vi "適應性控制_多頻率追蹤DAQmx_V4(實際控制).vi"() -> ()   [LabVIEW 2010]
uses:
  <vilib>/DAQmx/write.llb/DAQmx Write (Analog DBL 1Chan 1Samp).vi
  <vilib>/DAQmx/read.llb/DAQmx Read (Analog DBL 1Chan 1Samp).vi
  <vilib>/DAQmx/create/channels.llb/DAQmx Create Channel (AI-Voltage-Basic).vi
  <vilib>/DAQmx/configure/timing.llb/DAQmx Timing (Sample Clock).vi
  <vilib>/DAQmx/create/channels.llb/DAQmx Create Channel (AO-Voltage-Basic).vi
  <vilib>/daqmx/miscellaneous.llb/DAQmx Fill In Error Info.vi
panel:
  in  "DAQ output":tag
  in  "DAQ input":tag
  out "source out":string
  in  "理想初始頻率(Hz)":dbl=1.0
  in  "理想頻率數":i32=2
  out "當下誤差":dbl=0.1 format="%#_13g"
  out "實際輸入x(t)":dbl[][](graph)
  in  "頻率間距":dbl=1.0
  out "理想與FIR輸出":dbl[][](graph)
  out "誤差":dbl(graph)
  out "while平均運行時間":dbl
  out "收斂time":dbl
  out "各頻率誤差已達標準":bool
  in  "各頻率誤差低於多少亮燈":dbl=0.1 format="%#_13g"
  out "權重(w)":dbl[](array[numeric])
  in  "理想振幅":dbl=0.5
  in  "理想直流偏移":dbl
  in  "理想相位(deg)":dbl
  in  "收斂係數":dbl=0.0001
  in  "order":i32=150
  in  "取樣頻率":dbl=150.0 min=1.0 max=10000.0 step=1.0
  in  "stop":bool
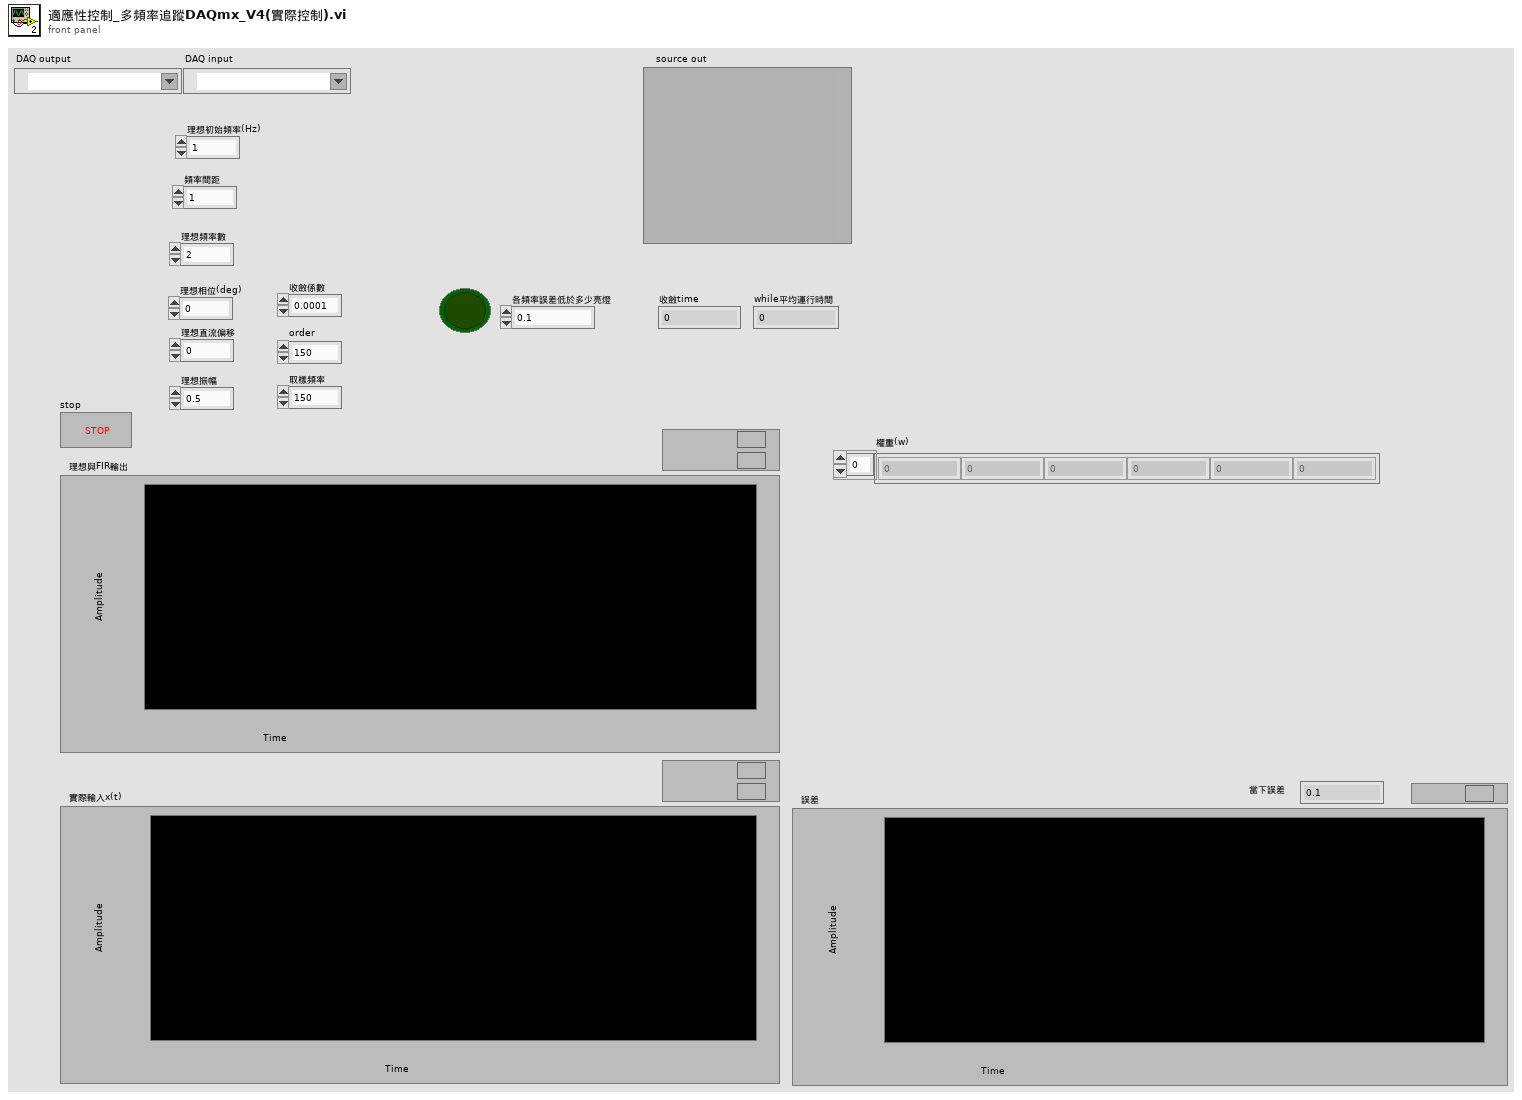
[diagram p1: front panel]
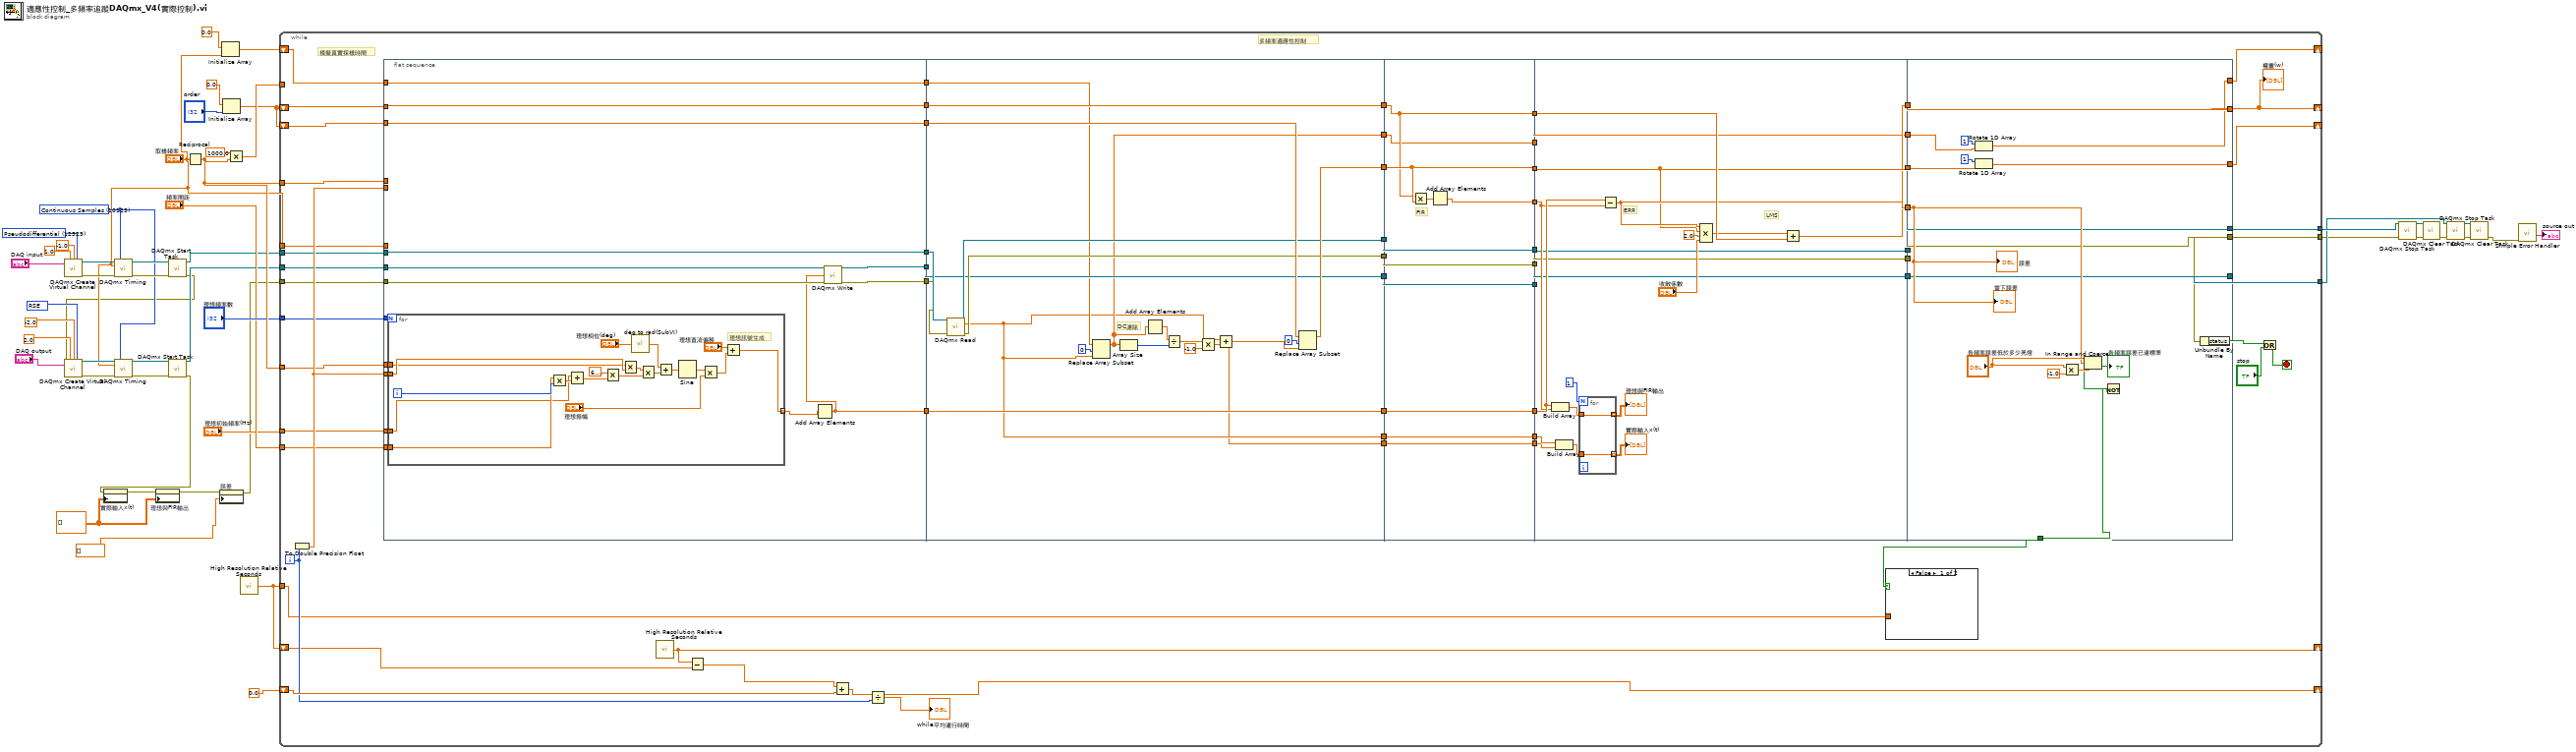
[diagram p0: block diagram]
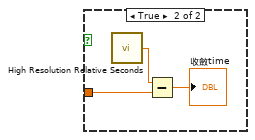
[diagram p2: hidden frame]
diagram:
  w23 = 10123 items=["Finite Samples"=10178, "Continuous Samples"=10123, "Hardware Timed Single Point"=12522] ("sample mode")
  w26 = 10083 items=["Default"=-1, "RSE"=10083, "Differential"=10106, "Pseudodifferential"=12529] ("output terminal configuration")
  w27 = 12529 items=["default"=-1, "RSE"=10083, "NRSE"=10078, "Differential"=10106, "Pseudodifferential"=12529] ("input terminal configuration")
  w9 = dbl[][] [] ("History Data")
  n1 = call-poly <vilib>:"DAQmx Create Virtual Channel.vi"("maximum value"=1.0, "minimum value"=-1.0, "input terminal configuration"=w27, "physical channels"="DAQ input") -> ("task out"=w36:refnum<k21>, "error out"=w32:errorcluster)  [unwired: 10 in]
  n2 = call-poly <vilib>:"DAQmx Timing.vi"("task/channels in"=w36, "sample mode"=w23, "rate"="取樣頻率", "error in"=w32) -> ("task out"=w35:refnum<k21>, "error out"=w33:errorcluster)  [unwired: 10 in]
  n3 = call <vilib>:"DAQmx Start Task.vi"("task/channels in"=w35, "error in"=w33) -> ("task out"=w34:refnum<k21>, "error out"=w8:errorcluster)  [unwired: 12 in]
  n4 = call-poly <vilib>:"DAQmx Create Virtual Channel.vi"("maximum value"=2.0, "minimum value"=-2.0, "output terminal configuration"=w26, "physical channels"="DAQ output", "error in"=w8) -> ("task out"=w28:refnum<k21>, "error out"=w31:errorcluster)  [unwired: 9 in]
  n5 = call-poly <vilib>:"DAQmx Timing.vi"("task/channels in"=w28, "sample mode"=w23, "rate"="取樣頻率", "error in"=w31) -> ("task out"=w29:refnum<k21>, "error out"=w30:errorcluster)  [unwired: 10 in]
  n6 = call <vilib>:"DAQmx Start Task.vi"("task/channels in"=w29, "error in"=w30) -> ("task out"=w22:refnum<k21>, "error out"=w5:errorcluster)  [unwired: 12 in]
  n7 = property on="實際輸入x(t)" class="WFChart (strict)"(error in=w5, "History Data"=w9) -> (error out=w43:errorcluster)  [unwired: 1 in, 1 out]
  n8 = property on="理想與FIR輸出" class="WFChart (strict)"(error in=w43, "History Data"=w9) -> (error out=w44:errorcluster)  [unwired: 1 in, 1 out]
  n9 = Reciprocal(x="取樣頻率") -> (1/x=w49:dbl)
  n10 = property on="誤差" class="WFChart (strict)"(error in=w44, "History Data"=dbl[] []) -> (error out=w4:errorcluster)  [unwired: 1 in, 1 out]
  n11 = Initialize Array(0.0 ("element"), "取樣頻率") -> (w10:dbl[])
  n12 = Initialize Array(0.0 ("element"), "order") -> (w40:dbl[])
  n13 = Multiply(x=1000.0, y=w49) -> (x*y=w47:dbl)
  n14 = call <vilib>:"High Resolution Relative Seconds.vi"() -> ("relative seconds"=w46:dbl)
  n15 = while {
    shift-right: [w86] -> _
    shift-left: w40 -> [w113]
    shift-right: [w101] -> _
    shift-left: w40 -> [w109]
    tunnel: w49 -> [w98]
    tunnel: w49 -> [w97]
    tunnel: w47 -> [_]
    tunnel: w46 -> [w89]
    shift-right: [w90] -> _
    shift-left: w46 -> [w88]
    shift-right: [w91] -> _
    shift-left: 0.0 -> [w93]
    tunnel: "理想頻率數" -> [w85]
    tunnel: "頻率間距" -> [w84]
    tunnel: "理想初始頻率(Hz)" -> [w83]
    tunnel: "取樣頻率" -> [w82]
    tunnel: w34 -> [w81]
    tunnel: w22 -> [w80]
    tunnel: w4 -> [w79]
    tunnel: [w52] -> w7
    tunnel: [w66] -> w19
    tunnel: [w65] -> w18
    shift-right: [w58] -> _
    shift-left: w10 -> [w60]
    i -> [w92]
    stop <- w63 stop-if-true
    # "模擬真實採樣時間"
    # "多頻率適應性控制"
    n16 = To Double Precision Float(number=w92) -> (double precision float=w107:dbl)
    n17 = flat-sequence {
      tunnel: w107 -> [_]
      tunnel: [w132] -> w114
      tunnel: w113 -> [w132]
      tunnel: [w131] -> w110
      tunnel: w109 -> [w131]
      tunnel: w107 -> [w130]
      tunnel: [w122] -> w104
      tunnel: w98 -> [_]
      tunnel: w97 -> [w129]
      tunnel: w85 -> [w128]
      tunnel: w84 -> [w127]
      tunnel: w83 -> [w126]
      tunnel: w82 -> [_]
      tunnel: w81 -> [w121]
      tunnel: w80 -> [w124]
      tunnel: w79 -> [w123]
      tunnel: [w121] -> w78
      tunnel: [w120] -> w77
      tunnel: [w119] -> w70
      tunnel: w60 -> [w118]
      tunnel: [w118] -> w59
      tunnel: w114 -> [w168]
      tunnel: [w171] -> w112
      tunnel: [w170] -> w111
      tunnel: w110 -> [w170]
      tunnel: [w169] -> w105
      tunnel: w104 -> [w169]
      tunnel: w78 -> [w166]
      tunnel: w77 -> [w153]
      tunnel: [w165] -> w76
      tunnel: [w164] -> w73
      tunnel: [w163] -> w71
      tunnel: w70 -> [w163]
      tunnel: [w155] -> w62
      tunnel: w59 -> [w157]
      tunnel: [w156] -> w57
      tunnel: [w154] -> w53
      tunnel: w112 -> [w174]
      tunnel: w111 -> [w173]
      tunnel: [w173] -> w108
      tunnel: [w182] -> w106
      tunnel: w105 -> [w182]
      tunnel: [w181] -> w103
      tunnel: [w174] -> w102
      tunnel: w76 -> [w179]
      tunnel: [w179] -> w75
      tunnel: w73 -> [w178]
      tunnel: [w178] -> w72
      tunnel: w71 -> [w177]
      tunnel: [w177] -> w69
      tunnel: w62 -> [w176]
      tunnel: [w176] -> w61
      tunnel: w57 -> [w172]
      tunnel: [w172] -> w56
      tunnel: [w175] -> w54
      tunnel: w53 -> [w175]
      tunnel: w108 -> [w202]
      tunnel: w106 -> [w193]
      tunnel: w103 -> [w192]
      tunnel: w102 -> [w197]
      tunnel: [w194] -> w100
      tunnel: [w197] -> w99
      tunnel: [w198] -> w96
      tunnel: w75 -> [w191]
      tunnel: [w191] -> w74
      tunnel: w72 -> [w189]
      tunnel: w69 -> [w190]
      tunnel: [w190] -> w68
      tunnel: [w189] -> w67
      tunnel: w61 -> [w187]
      tunnel: w56 -> [w188]
      tunnel: [w188] -> w55
      tunnel: w54 -> [w186]
      tunnel: [w220] -> w101
      tunnel: w100 -> [w220]
      tunnel: w99 -> [w213]
      tunnel: [w219] -> w86
      tunnel: w96 -> [w211]
      tunnel: [w215] -> w87
      tunnel: w74 -> [w210]
      tunnel: [w210] -> w52
      tunnel: w68 -> [w208]
      tunnel: w67 -> [w209]
      tunnel: [w209] -> w66
      tunnel: [w208] -> w65
      tunnel: [w205] -> w58
      tunnel: w55 -> [w206]
      frame #0 {
        n18 = for {
          N: w128 -> [_]
          tunnel: w130 -> [w151]
          tunnel: [w150] -> w125 mode=indexing
          tunnel: w129 -> [w149]
          tunnel: w127 -> [w135]
          tunnel: w126 -> [w134]
          i -> [w136]
          # "理想訊號生成"
          n19 = Multiply(x=w135, y=w136) -> (x*y=w137:dbl)
          n20 = Add(x=w134, y=w137) -> (x+y=w133:dbl)
          n21 = Multiply(x=6.283185307179586, y=w133) -> (x*y=w146:dbl)
          n22 = Multiply(x=w149, y=w151) -> (x*y=w139:dbl)
          n23 = call "deg to rad(SubVI).vi"("Degree"="理想相位(deg)") -> ("Radian"=w143:dbl)
          n24 = Multiply(x=w139, y=w146) -> (x*y=w147:dbl)
          n25 = Add(x=w143, y=w147) -> (x+y=w148:dbl)
          n26 = Sine(x=w148) -> (sin(x)=w144:dbl)
          n27 = Multiply(x=w144, y="理想振幅") -> (x*y=w145:dbl)
          n28 = Add(x="理想直流偏移", y=w145) -> (x+y=w150:dbl)
        }
        n29 = Add Array Elements(numeric array=w125) -> (sum=w122:dbl)
        n30 = call-poly <vilib>:"DAQmx Write.vi"("task/channels in"=w124, "data"=w122, "error in"=w123) -> ("task out"=w119:refnum<k21>, "error out"=w120:errorcluster)  [unwired: 10 in, 1 out]
      }
      frame #1 {
        # "DC濾除"
        n31 = call-poly <vilib>:"DAQmx Read.vi"("task/channels in"=w166, "error in"=w153) -> ("task out"=w164:refnum<k21>, "data"=w155:dbl, "error out"=w165:errorcluster)  [unwired: 11 in]
        n32 = Replace Array Subset(array=w157, new element=w155, index=0) -> (w156:dbl[])
        n33 = Array Size(array=w156) -> (size(s)=w160:i32)
        n34 = Add Array Elements(numeric array=w156) -> (sum=w159:dbl)
        n35 = Divide(x=w159, y=w160) -> (x/y=w161:dbl)
        n36 = Multiply(x=w161, y=-1.0) -> (x*y=w162:dbl)
        n37 = Add(x=w155, y=w162) -> (x+y=w154:dbl)
        n38 = Replace Array Subset(array=w168, new element=w154, index=0) -> (w171:dbl[])
      }
      frame #2 {
        # "FIR"
        n39 = Multiply(x=w173, y=w174) -> (x*y=w180:dbl[])
        n40 = Add Array Elements(numeric array=w180) -> (sum=w181:dbl)
      }
      frame #3 {
        # "LMS"
        # "ERR"
        n41 = Build Array(w193, w192) -> (w201:dbl[])
        n42 = Build Array(w187, w186) -> (w185:dbl[])
        n43 = for {
          N: 1 -> [_]
          tunnel: [w204] -> w195 mode=indexing
          tunnel: w201 -> [w204]
          tunnel: w185 -> [w203]
          tunnel: [w203] -> w184 mode=indexing
        }
        "理想與FIR輸出" <- w195
        "實際輸入x(t)" <- w184
        n44 = Subtract(x=w193, y=w192) -> (x-y=w198:dbl)
        n45 = Compound Arithmetic op=MULTIPLY(w198, w197, 2.0, "收斂係數") -> (w196:dbl[])
        n46 = Add(x=w196, y=w202) -> (x+y=w194:dbl[])
      }
      frame #4 {
        n47 = Rotate 1D Array(1:w206, 2:1 ("n")) -> (0:w205:dbl[])
        n48 = Rotate 1D Array(1:w213, 2:1 ("n")) -> (0:w219:dbl[])
        n49 = Multiply(x="各頻率誤差低於多少亮燈", y=-1.0) -> (x*y=w216:dbl)
        n50 = In Range and Coerce(upper limit="各頻率誤差低於多少亮燈", x=w211, lower limit=w216) -> (In Range?=w212:bool)  [unwired: 1 out]
        "各頻率誤差已達標準" <- w212
        n51 = Not(x=w212) -> (.not. x?=w215:bool)
        "誤差" <- w211
        "當下誤差" <- w211
      }
    }
    n52 = call <vilib>:"High Resolution Relative Seconds.vi"() -> ("relative seconds"=w90:dbl)
    n53 = Subtract(x=w90, y=w88) -> (x-y=w95:dbl)
    n54 = Add(x=w95, y=w93) -> (x+y=w91:dbl)
    n55 = Divide(x=w91, y=w92) -> (x/y=→"while平均運行時間":dbl)
    n56 = case shown="False" w87 {
      tunnel: w89 -> [_ w115]
      frame False {
      }
      frame True {
        n57 = call <vilib>:"High Resolution Relative Seconds.vi"() -> ("relative seconds"=w117:dbl)
        n58 = Subtract(x=w117, y=w115) -> (x-y=→"收斂time":dbl)
      }
    }
    n59 = Unbundle By Name(w52) -> ("status"=w51:bool)
    n60 = Or(x=w51, y="stop") -> (x .or. y?=w63:bool)
    "權重(w)" <- w101
  }
  n61 = call <vilib>:"DAQmx Stop Task.vi"("task/channels in"=w19, "error in"=w7) -> ("task out"=w21:refnum<k21>, "error out"=w20:errorcluster)  [unwired: 12 in]
  n62 = call <vilib>:"DAQmx Clear Task.vi"("task in"=w21, "error in"=w20) -> ("error out"=w6:errorcluster)  [unwired: 13 in]
  n63 = call <vilib>:"DAQmx Stop Task.vi"("task/channels in"=w18, "error in"=w6) -> ("task out"=w16:refnum<k21>, "error out"=w17:errorcluster)  [unwired: 12 in]
  n64 = call <vilib>:"DAQmx Clear Task.vi"("task in"=w16, "error in"=w17) -> ("error out"=w3:errorcluster)  [unwired: 13 in]
  n65 = call <vilib>:"Simple Error Handler.vi"("error in (no error)"=w3) -> ("source out"=→"source out":string)  [unwired: 4 in, 4 out]
